vi "subStage_MoveLimitation.vi"(7 "Stage-Ctrl":T1={"Console"={"L"=FALSE, "R"=FALSE, "FWD"=FALSE, "BACK"=FALSE}, "Step Width [mm]"=1.0, "Destination [mm]"=[6.0, 7.0], "Move "=FALSE} {"Destination [mm]" format="%_6g"; "Step Width [mm]" min=0.0 format="%_6f"}, 11 "Stage setting":T2={"Baudrate"=57600, "COM Port"="COM10", "Xmax"=118.5, "Xmin"=15.0, "Ymax"=76.5, "Ymin"=12.2}) -> (3 "Allow?":bool)   [LabVIEW 2015]
panel:
  # "This VI is used for limiting the zone of movement of stage in case of collide objectives."
  # "X"
  # "Y"
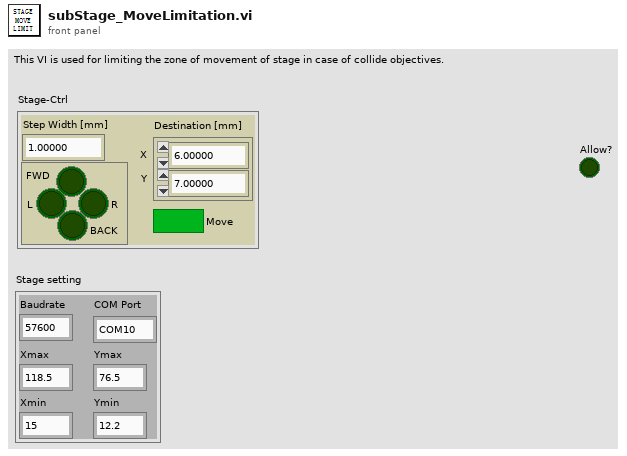
[diagram p1: front panel]
types:
  T1 = cluster{"Console":cluster{"L":bool, "R":bool, "FWD":bool, "BACK":bool}, "Step Width [mm]":dbl, "Destination [mm]":dbl[], "Move ":bool}
  T2 = cluster{"Baudrate":i32, "COM Port":string, "Xmax":dbl, "Xmin":dbl, "Ymax":dbl, "Ymin":dbl}
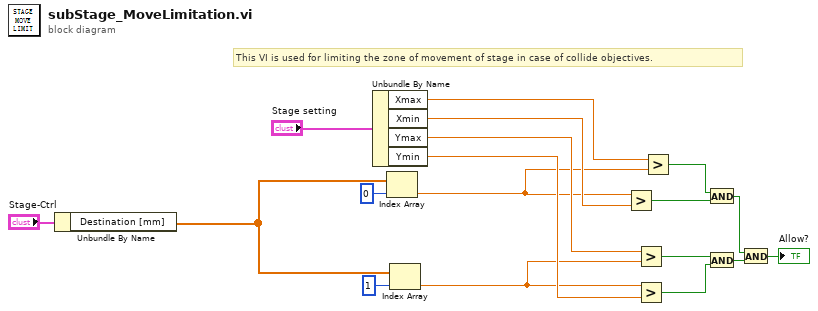
[diagram p0: block diagram]
diagram:
  # "This VI is used for limiting the zone of movement of stage in case of collide objectives."
  n1 = Unbundle By Name("Stage-Ctrl") -> ("Destination [mm]"=w1:dbl[])
  n2 = Unbundle By Name("Stage setting") -> ("Xmax"=w10:dbl, "Xmin"=w9:dbl, "Ymax"=w8:dbl, "Ymin"=w7:dbl)
  n3 = Index Array(array=w1, index=0) -> (element=w4:dbl)
  n4 = Index Array(array=w1, index=1) -> (element=w2:dbl)
  n5 = Greater?(x=w4, y=w9) -> (0:w13:bool)
  n6 = Greater?(x=w8, y=w2) -> (0:w14:bool)
  n7 = Greater?(x=w2, y=w7) -> (0:w15:bool)
  n8 = Greater?(x=w10, y=w4) -> (0:w16:bool)
  n9 = And(x=w16, y=w13) -> (x .and. y?=w17:bool)
  n10 = And(x=w14, y=w15) -> (x .and. y?=w18:bool)
  n11 = And(x=w17, y=w18) -> (x .and. y?=→"Allow?":bool)
